vi "Main.vi"() -> ()   [LabVIEW 2026]
doc: "This template is for the Queued Message Handler design pattern.\n\nThe Event Handling Loop generates messages based on user interface actions.\n\nThe Message Handling Loop processes messages generated by the Event Handling Loop, or by other messages. The messages are string values, so new messages can be added easily to the Message Cases case structure in the Message Handling Loop. Each message cluster can also provide an optional value for Message Data, which is a variant that can be converted to whatever message-specific data is required."
uses:
  controls/UI Data.ctl
  controls/State_Enum.ctl
  support/Message Queue/Enqueue Message (Single).vi
  <vilib>/Utility/error.llb/Error Cluster From Error Code.vi
  <vilib>/ErrorRing/Error Ring.xnode
  support/Message Queue/Message Queue.lvlib
  support/User Event - Stop/User Event - Stop.lvlib
panel:
  in  "Mode":bool
  out "Panel":cluster{"On LED":bool, "Buzzer":bool}
  in  "Door Sensor":bool
  out "Recipes":string[][](array[string])
  in  "Key Pad":T1
  out "Display":string="00:00"
  in  "Exit":bool
  # "Manual"
  # "Recipe"
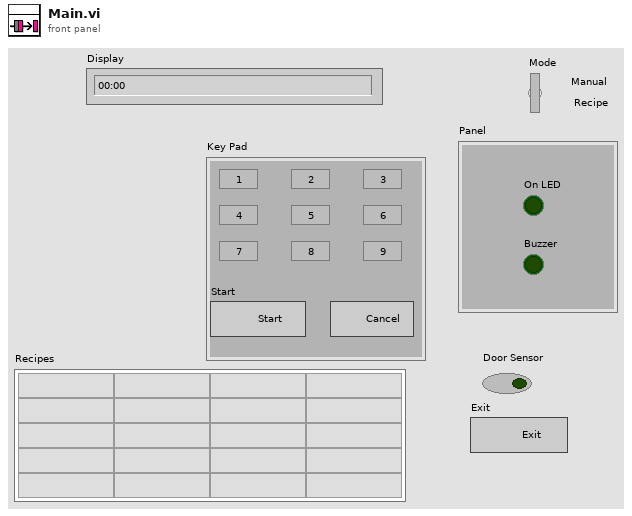
[diagram p1: front panel]
types:
  T1 = cluster{"1":bool, "2":bool, "3":bool, "4":bool, "5":bool, "6":bool, "7":bool, "8":bool, "9":bool, "Start":bool, "Cancel":bool}
  T2 = typedef "UI Data.ctl" = cluster{"Mode":bool, "Display":string, "Target Time ":dbl, "Data Display Ref":refnum<vi>, "Exit Button Ref":refnum<vi>, "Recipe":i32, "Step":i32, "Door Sensor":bool}
  T3 = typedef "Message Queue.lvlib/All Message Queues.ctl" = cluster{"UI":refnum<queue>}
  T4 = typedef "State_Enum.ctl" = enum16{"Complete", "Run", "Idle"}
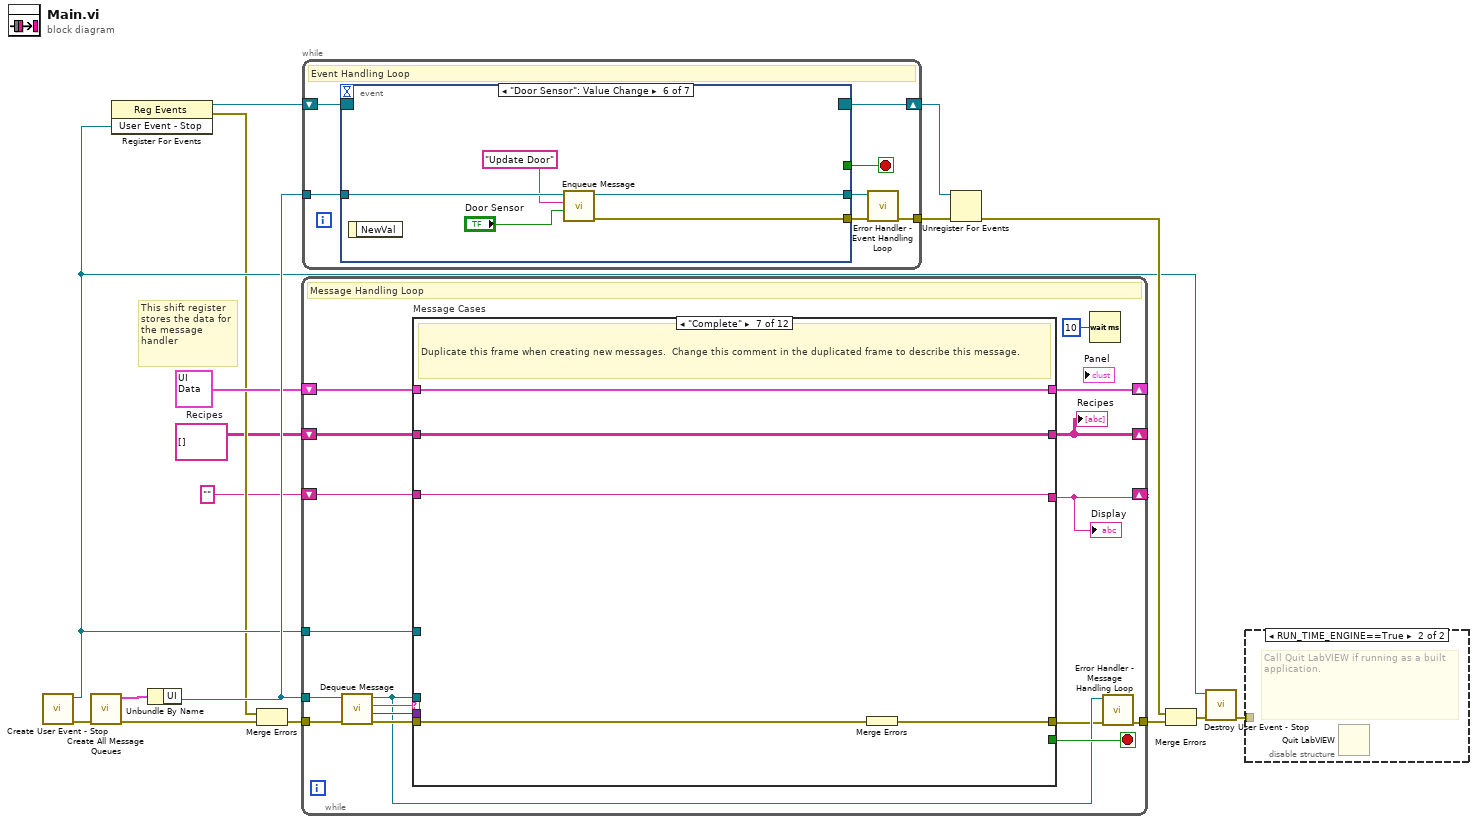
[diagram p0: block diagram]
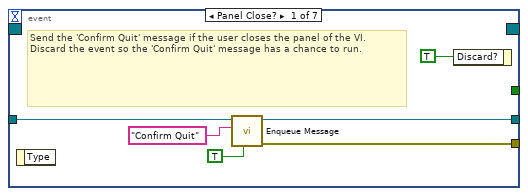
[diagram p3: hidden frame]
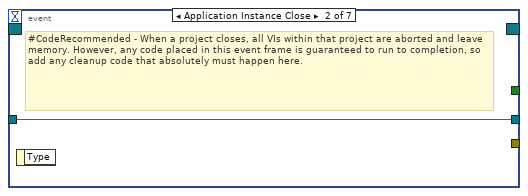
[diagram p4: hidden frame]
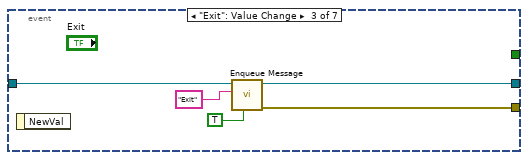
[diagram p5: hidden frame]
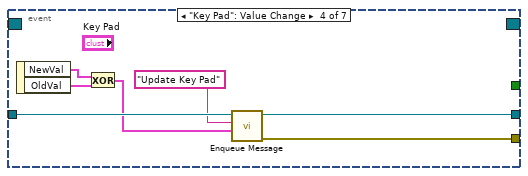
[diagram p6: hidden frame]
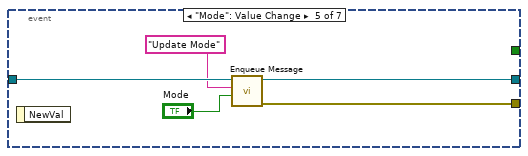
[diagram p7: hidden frame]
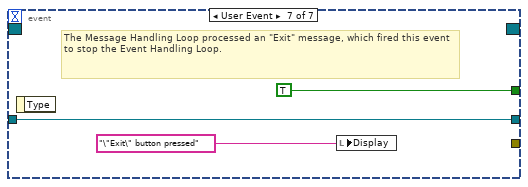
[diagram p8: hidden frame]
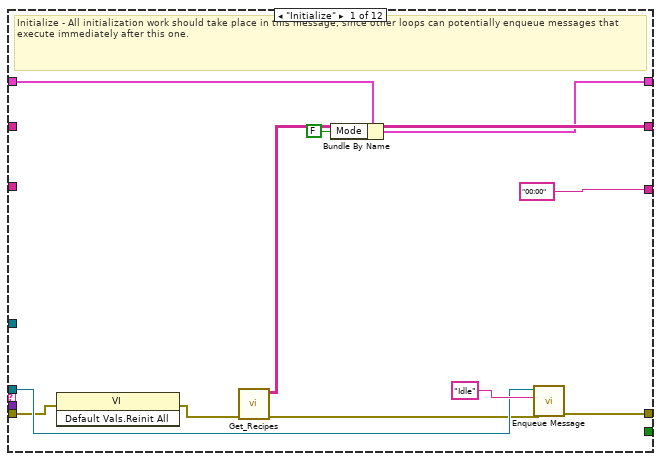
[diagram p9: hidden frame]
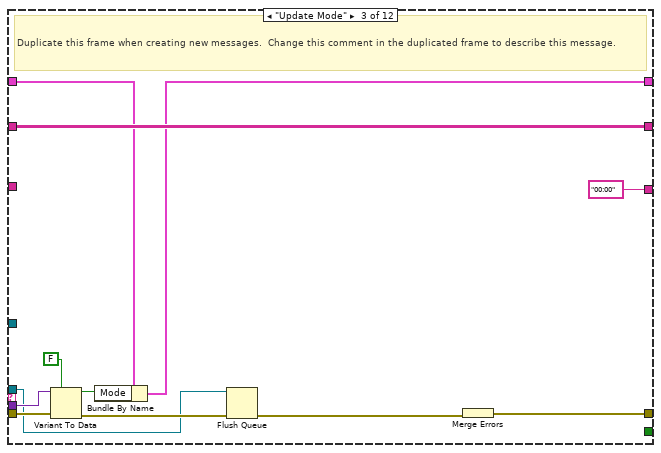
[diagram p11: hidden frame]
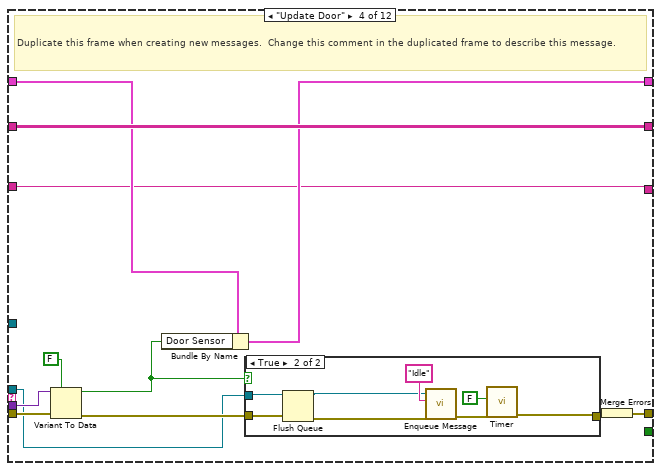
[diagram p12: hidden frame]
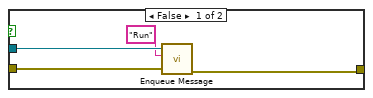
[diagram p13: hidden frame]
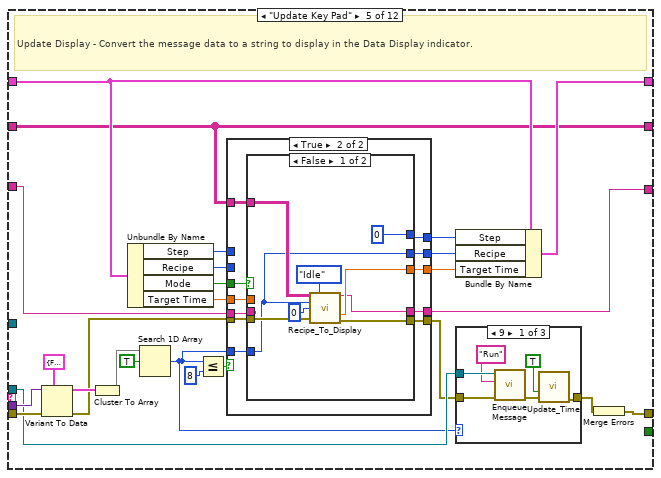
[diagram p14: hidden frame]
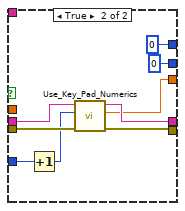
[diagram p16: hidden frame]
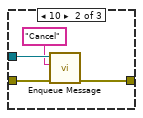
[diagram p17: hidden frame]
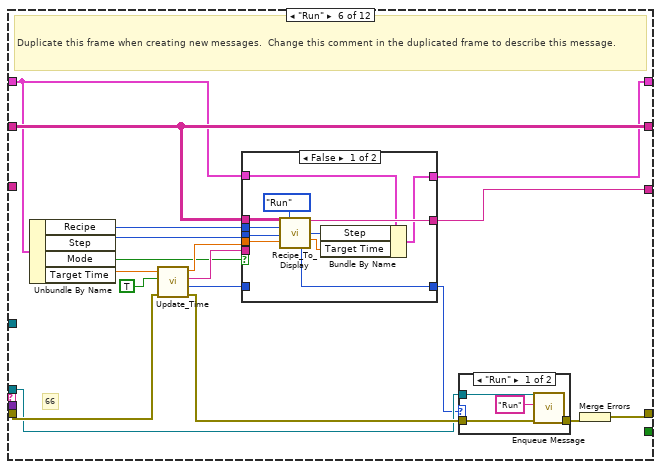
[diagram p19: hidden frame]
diagram:
  w2 = string[][] []  # Recipes
  # "This shift register stores the data for the message handler"
  n1 = call "Create User Event - Stop.vi"() -> ("error out"=w13:errorcluster, "User Event - Stop"=w5:refnum<user-event>)  [unwired: 10 in]
  n2 = call "Create All Message Queues.vi"("error in (no error)"=w13) -> ("error out"=w17:errorcluster, "Message Queues out"=w16:T3)  [unwired: 9 in]
  n3 = register-events(w5) -> (reference out=w6:refnum<event-registration>, error out=w3:errorcluster)  [unwired: 2 in]
  n4 = Unbundle By Name(w16) -> ("UI"=w14:refnum<queue>)
  n5 = Merge Errors(w3, w17) -> (w4:errorcluster)
  n6 = while {
    tunnel: w14 -> [w26]
    shift-right: [w33] -> _
    shift-left: T2 {"Mode"=FALSE, "Display"="", "Target Time "=0.0, "Data Display Ref"=refnum, "Exit Button Ref"=refnum, "Recipe"=0, "Step"=0, "Door Sensor"=FALSE} ("Data Cluster") -> [w34]
    tunnel: w5 -> [w31]
    tunnel: w4 -> [w30]
    tunnel: [w24] -> w15
    shift-right: [w22] -> _
    shift-left: w2 -> [w21]
    shift-right: [w19] -> _
    shift-left: "" ("String out") -> [w20]
    stop <- w32 stop-if-true
    # "Message Handling Loop"
    n7 = call "Dequeue Message.vi"("error in (no error)"=w30, "Message Queue"=w26) -> ("error out"=w29:errorcluster, "Message Data"=w27:variant, "Message"=w28:string, "dup Message Queue"=w25:refnum<queue>)  [unwired: 6 in]
    n8 = case "Message Cases" shown="\"Complete\"" w28 {
      selector: w28 -> [_ _ _ _ _ _ _ _ _ _ _ w240]
      tunnel: w25 -> [w43 _ w50 w63 w96 w169 _ _ w215 _ w237 _]
      tunnel: w29 -> [w41 w49 w59 w71 w110 w173 w201 w210 w219 w224 w230 _]
      tunnel: [w45 w49 w61 w73 w111 w174 w199 w204 w217 w222 w233 w241] -> w23
      tunnel: w34 -> [w37 w48 w57 w69 w101 w158 w200 w209 w218 w223 w236 w242]
      tunnel: [w36 w48 w55 w68 w102 w159 w200 w209 w218 w223 w236 w242] -> w33
      tunnel: [_ _ _ _ _ _ _ _ _ _ TRUE _] -> w32
      tunnel: w27 -> [_ _ w54 w67 w109 _ _ w208 _ _ w227 _]
      tunnel: w31 -> [_ _ _ _ _ _ _ _ _ _ w232 _]
      tunnel: [w39 w47 w60 w72 w93 w168 w198 w203 w212 w221 w226 w239] -> w22
      tunnel: w21 -> [_ w47 w60 w72 w93 w168 w198 w203 w212 w221 w226 w239]
      tunnel: ["00:00" ("Initial Message") w46 "00:00" ("String out") w66 w94 w157 w197 w202 w211 w220 w225 w238] -> w19
      tunnel: w20 -> [_ w46 _ w66 w103 _ w197 w202 w211 w220 w225 w238]
      frame "Initialize" {
        # "Initialize - All initialization work should take place in this message, since other loops can potentially enqueue messages that execute immediately after this one."
        n9 = invoke class="VI" method="Default Vals.Reinit All"(error in=w41) -> (error out=w42:errorcluster)  [unwired: 2 in, 2 out]
        n10 = call "Get_Recipes.vi"("error in (no error)"=w42) -> ("error out"=w40:errorcluster, "Recipes"=w39:string[][])  [unwired: 9 in]
        n11 = Bundle By Name(cluster=w37, "Mode"=FALSE) -> (w36:T2)
        n12 = call-poly "Enqueue Message.vi"("error in (no error)"=w40, "Message"="Idle", "Message Queue"=w43) -> ("error out"=w45:errorcluster)  [unwired: 7 in, 1 out]
      }
      frame "Idle" {
      }
      frame "Update Mode" {
        # "Duplicate this frame when creating new messages.  Change this comment in the duplicated frame to describe this message."
        n13 = Variant To Data(error in=w59, type=FALSE, Variant=w54) -> (data=w56:bool, error out=w52:errorcluster)
        n14 = Bundle By Name(cluster=w57, "Mode"=w56) -> (w55:T2)
        n15 = Flush Queue(queue=w50, error in (no error)=w52) -> (error out=w51:errorcluster)  [unwired: 2 out]
        n16 = Merge Errors(w51) -> (w61:errorcluster)
      }
      frame "Update Door" {
        # "Duplicate this frame when creating new messages.  Change this comment in the duplicated frame to describe this message."
        n17 = Variant To Data(error in=w71, type=FALSE, Variant=w67) -> (data=w62:bool, error out=w64:errorcluster)
        n18 = Bundle By Name(cluster=w69, "Door Sensor"=w62) -> (w68:T2)
        n19 = case shown="True" w62 {
          tunnel: [w76 w79] -> w65
          tunnel: w64 -> [w77 w84]
          tunnel: w63 -> [w75 w82]
          frame False {
            n20 = call-poly "Enqueue Message.vi"("error in (no error)"=w77, "Message"="Run", "Message Queue"=w75) -> ("error out"=w76:errorcluster)  [unwired: 7 in, 1 out]
          }
          frame True {
            n21 = Flush Queue(queue=w82, error in (no error)=w84) -> (queue out=w81:refnum<queue>, error out=w83:errorcluster)  [unwired: 1 out]
            n22 = call-poly "Enqueue Message.vi"("error in (no error)"=w83, "Message"="Idle", "Message Queue"=w81) -> ("error out"=w80:errorcluster)  [unwired: 7 in, 1 out]
            n23 = call "Timer.vi"("error in (no error)"=w80, "Advance?"=FALSE) -> ("error out"=w79:errorcluster)  [unwired: 6 in, 3 out]
          }
        }
        n24 = Merge Errors(w65) -> (w73:errorcluster)
      }
      frame "Update Key Pad" {
        # "Update Display - Convert the message data to a string to display in the Data Display indicator."
        n25 = Variant To Data(error in=w110, type=T1 {"1"=FALSE, "2"=FALSE, "3"=FALSE, "4"=FALSE, "5"=FALSE, "6"=FALSE, "7"=FALSE, "8"=FALSE, "9"=FALSE, "Start"=FALSE, "Cancel"=FALSE} ("x .xor. y?"), Variant=w109) -> (data=w107:T1, error out=w104:errorcluster)
        n26 = Cluster To Array(cluster=w107) -> (array=w106:bool[])
        n27 = Unbundle By Name(w101) -> ("Step"=w87:i32, "Recipe"=w86:i32, "Mode"=w100:bool, "Target Time"=w91:dbl)
        n28 = Search 1D Array(1D array=w106, element=TRUE) -> (index of element=w88:i32)  [unwired: 1 in]
        n29 = Less Or Equal?(x=w88, y=8) -> (x <= y?=w89:bool)
        n30 = case shown="True" w89 {
          tunnel: w104 -> [w116 w127]
          tunnel: w103 -> [w115 w126]
          tunnel: w100 -> [_ w125]
          tunnel: [w112 w124] -> w99
          tunnel: [w113 w123] -> w98
          tunnel: [w116 w122] -> w95
          tunnel: [w115 w121] -> w94
          tunnel: w93 -> [_ w120]
          tunnel: [w114 w119] -> w92
          tunnel: w91 -> [w114 w118]
          tunnel: w88 -> [_ w117]
          tunnel: w87 -> [w113 _]
          tunnel: w86 -> [w112 _]
          frame False {
          }
          frame True {
            n31 = case shown="False" w125 {
              tunnel: w127 -> [w135 w140]
              tunnel: w126 -> [_ w139]
              tunnel: [w128 0 ("upper limit")] -> w124
              tunnel: [0 0] -> w123
              tunnel: [w134 w143] -> w122
              tunnel: [w129 w142] -> w121
              tunnel: w120 -> [w133 _]
              tunnel: [w131 w141] -> w119
              tunnel: w118 -> [_ _]
              tunnel: w117 -> [w128 w137]
              frame False {
                n32 = call "Recipe_To_Display.vi"("Recipes"=w133, "State In"=State_Enum."Idle" ("Enum"), "Recipe"=w128, "Step In"=0 ("Step"), "error in (no error)"=w135) -> ("Display Out"=w129:string, "Target Time"=w131:dbl, "error out"=w134:errorcluster)  [unwired: 6 in, 2 out]
              }
              frame True {
                n33 = Increment(x=w137) -> (x+1=w138:i32)
                n34 = call "Use_Key_Pad_Numerics.vi"("error in (no error)"=w140, "Key Pad"=w138, "Display in"=w139) -> ("error out"=w143:errorcluster, "Elaspsed Time"=w141:dbl, "Display out"=w142:string)  [unwired: 6 in]
              }
            }
          }
        }
        n35 = Bundle By Name(cluster=w101, "Step"=w98, "Recipe"=w99, "Target Time"=w92) -> (w102:T2)
        n36 = case shown="9" w88 {
          tunnel: w96 -> [w151 w155 _]
          tunnel: [w148 w153 w156] -> w97
          tunnel: w95 -> [w146 w152 w156]
          frame 9 {
            n37 = call-poly "Enqueue Message.vi"("error in (no error)"=w146, "Message"="Run", "Message Queue"=w151) -> ("error out"=w149:errorcluster)  [unwired: 7 in, 1 out]
            n38 = call "Update_Time.vi"("error in (no error)"=w149, "Reset?"=TRUE) -> ("error out"=w148:errorcluster)  [unwired: 6 in, 3 out]
          }
          frame 10 {
            n39 = call-poly "Enqueue Message.vi"("error in (no error)"=w152, "Message"="Cancel", "Message Queue"=w155) -> ("error out"=w153:errorcluster)  [unwired: 7 in, 1 out]
          }
          frame 11, Default {
          }
        }
        n40 = Merge Errors(w97) -> (w111:errorcluster)
      }
      frame "Run" {
        # "66"
        # "Duplicate this frame when creating new messages.  Change this comment in the duplicated frame to describe this message."
        n41 = Unbundle By Name(w158) -> ("Recipe"=w167:i32, "Step"=w166:i32, "Mode"=w163:bool, "Target Time"=w172:dbl)
        n42 = call "Update_Time.vi"("error in (no error)"=w173, "Advance?"=TRUE, "Target Time"=w172) -> ("error out"=w171:errorcluster, "State"=w162:T4, "Display Out"=w164:string, "Time Remaining"=w165:dbl)  [unwired: 5 in]
        n43 = case shown="False" w163 {
          tunnel: w168 -> [w185 _]
          tunnel: w167 -> [w184 _]
          tunnel: w166 -> [w183 _]
          tunnel: w165 -> [w182 _]
          tunnel: [w180 w188] -> w157
          tunnel: w164 -> [_ w188]
          tunnel: w162 -> [_ w187]
          tunnel: [w179 w187] -> w161
          tunnel: [w175 w186] -> w159
          tunnel: w158 -> [w178 w186]
          frame False {
            n44 = call "Recipe_To_Display.vi"("Recipes"=w185, "State In"=State_Enum."Run" ("State"), "Recipe"=w184, "Step In"=w183, "Time Remaining"=w182) -> ("State Out"=w179:T4, "Display Out"=w180:string, "Step Out"=w177:i32, "Target Time"=w176:dbl)  [unwired: 6 in, 1 out]
            n45 = Bundle By Name(cluster=w178, "Step"=w177, "Target Time"=w176) -> (w175:T2)
          }
          frame True {
          }
        }
        n46 = case shown="\"Run\"" w161 {
          tunnel: w171 -> [w192 w196]
          tunnel: [w191 w195] -> w170
          tunnel: w169 -> [w189 w193]
          frame "Run" {
            n47 = call-poly "Enqueue Message.vi"("error in (no error)"=w192, "Message"="Run", "Message Queue"=w189) -> ("error out"=w191:errorcluster)  [unwired: 7 in, 1 out]
          }
          frame "Complete", Default {
            n48 = call-poly "Enqueue Message.vi"("error in (no error)"=w196, "Message"="Complete", "Message Queue"=w193) -> ("error out"=w195:errorcluster)  [unwired: 7 in, 1 out]
          }
        }
        n49 = Merge Errors(w170) -> (w174:errorcluster)
      }
      frame "Complete" {
        # "Duplicate this frame when creating new messages.  Change this comment in the duplicated frame to describe this message."
        n50 = Merge Errors(w201) -> (w199:errorcluster)
      }
      frame "Error" {
        # "Error - Display an error dialog. This message is sent by the \"Error Handler\" VIs at the end of other loops in this application."
        n51 = Variant To Data(error in=w210, type=errorcluster {"status"=FALSE, "code"=0, "source"=""} ("error constant"), Variant=w208) -> (data=w206:errorcluster, error out=w205:errorcluster)
        n52 = call <vilib>:"Simple Error Handler.vi"("error in (no error)"=w206) -> ()  [unwired: 4 in, 5 out]
        n53 = Merge Errors(w205) -> (w204:errorcluster)
      }
      frame "Confirm Quit" {
        # "#CodeNeeded - If you want to provide an \"Are you sure\" dialog (or some other notification) before the application exits, place that code here. This message is typically sent from a Panel Close? event."
        # "Confirm Quit - Message that can confirm whether or not the user wants to exit the application."
        n54 = call-poly "Enqueue Message.vi"("Priority Message? (F)"=TRUE, "error in (no error)"=w219, "Message"="Exit", "Message Queue"=w215) -> ("error out"=w216:errorcluster)  [unwired: 6 in, 1 out]
        n55 = Merge Errors(w216) -> (w217:errorcluster)
      }
      frame "---Copy This Frame---" {
        # "Duplicate this frame when creating new messages.  Change this comment in the duplicated frame to describe this message."
        n56 = Merge Errors(w224) -> (w222:errorcluster)
      }
      frame "Exit" {
        # "Stop the VI"
        # "Release the message queue reference"
        # "#CodeNeeded - Add any required cleanup code here. Note that if 'Exit' was called as a result of an error, an error dialog will be displayed. Add any custom error handling for an 'Exit' condition here as well."
        # "Exit - Exit the application."
        n57 = Variant To Data(type=errorcluster {"status"=FALSE, "code"=0, "source"=""} ("error constant"), Variant=w227) -> (data=w228:errorcluster)  [unwired: 1 in, 1 out]
        n58 = call <vilib>:"Simple Error Handler.vi"("error in (no error)"=w228) -> ()  [unwired: 4 in, 5 out]
        n59 = call "Fire User Event - Stop.vi"("User Event - Stop"=w232) -> ("error out"=w231:errorcluster)  [unwired: 10 in]
        n60 = Release Queue(queue=w237, error in (no error)=w230) -> (error out=w234:errorcluster)  [unwired: 1 in, 2 out]
        n61 = Merge Errors(w231, w234) -> (w233:errorcluster)
      }
      frame Default {
        # "'Default' case only runs if there is a message that isn't defined in any of the other cases.  Output a programming error."
        n62 = xnode "Error Ring"("parameter 0"=w240) -> ("error out"=w241:errorcluster)
      }
    }
    "Recipes" <- w22
    "Display" <- w19
    n63 = Wait (ms)(milliseconds to wait=u32 10) -> ()  [unwired: 1 out]
    n64 = call "Error Handler - Message Handling Loop.vi"("error in (no error)"=w23, "Message Queue"=w25) -> ("dup error in"=w24:errorcluster)  [unwired: 8 in, 1 out]
  }
  n65 = while {
    tunnel: w14 -> [w256]
    shift-right: [w254] -> w10
    shift-left: w6 -> [w255]
    tunnel: [w250] -> w7
    stop <- w252 stop-if-true
    # "Event Handling Loop"
    n66 = event shown="[5] \"Door Sensor\": Value Change" {
      selector: w255 -> [_ _ _ _ _ _ _]
      dyn-events: [_ _ _ _ _ _ _] -> w254
      timeout: _ -> [_ _ _ _ _ _ _]
      tunnel: [_ _ _ _ _ _ TRUE ("Discard?")] -> w252
      tunnel: w256 -> [w261 w263 w268 w273 w280 w285 w288]
      tunnel: [w260 _ w267 w271 w278 w283 _] -> w253
      tunnel: [w259 w263 w266 w272 w279 w284 w288] -> w251
      event Panel Close? {
        # "Send the 'Confirm Quit' message if the user closes the panel of the VI. Discard the event so the 'Confirm Quit' message has a chance to run."
        n67 = event-data() -> ()  [unwired: 1 in, 1 out]
        n68 = call-poly "Enqueue Message.vi"("Priority Message? (F)"=TRUE, "Message"="Confirm Quit", "Message Queue"=w261) -> ("error out"=w260:errorcluster, "dup Message Queue"=w259:refnum<queue>)  [unwired: 7 in]
        n69 = event-data("Discard?"=TRUE) -> ()  [unwired: 1 in, 1 out]
      }
      event Application Instance Close {
        # "#CodeRecommended - When a project closes, all VIs within that project are aborted and leave memory. However, any code placed in this event frame is guaranteed to run to completion, so add any cleanup code that absolutely must happen here."
        n70 = event-data() -> ()  [unwired: 1 in, 1 out]
      }
      event "Exit": Value Change {
        n71 = event-data() -> ()  [unwired: 1 in, 1 out]
        n72 = call-poly "Enqueue Message.vi"("Priority Message? (F)"=TRUE, "Message"="Exit", "Message Queue"=w268) -> ("error out"=w267:errorcluster, "dup Message Queue"=w266:refnum<queue>)  [unwired: 7 in]
      }
      event "Key Pad": Value Change {
        n73 = event-data() -> ("NewVal"=w275:T1, "OldVal"=w274:T1)  [unwired: 1 in]
        n74 = Exclusive Or(1:w274, 2:w275) -> (0:w269:T1)
        n75 = call-poly "Enqueue Message.vi"("Message Data"=w269, "Message"="Update Key Pad", "Message Queue"=w273) -> ("error out"=w271:errorcluster, "dup Message Queue"=w272:refnum<queue>)  [unwired: 7 in]
      }
      event "Mode": Value Change {
        n76 = event-data() -> ()  [unwired: 1 in, 1 out]
        n77 = call-poly "Enqueue Message.vi"("Message Data"="Mode", "Message"="Update Mode", "Message Queue"=w280) -> ("error out"=w278:errorcluster, "dup Message Queue"=w279:refnum<queue>)  [unwired: 7 in]
      }
      event "Door Sensor": Value Change {
        n78 = event-data() -> ()  [unwired: 1 in, 1 out]
        n79 = call-poly "Enqueue Message.vi"("Message Data"="Door Sensor", "Message"="Update Door", "Message Queue"=w285) -> ("error out"=w283:errorcluster, "dup Message Queue"=w284:refnum<queue>)  [unwired: 7 in]
      }
      event User Event {
        # "The Message Handling Loop processed an \"Exit\" message, which fired this event to stop the Event Handling Loop."
        n80 = event-data() -> ()  [unwired: 1 in, 1 out]
        n81 = local write "Display"("\"Exit\" button pressed" ("VI Stopped")) -> ()
      }
    }
    n82 = call "Error Handler - Event Handling Loop.vi"("error in (no error)"=w253, "Message Queue"=w251) -> ("dup error in"=w250:errorcluster)  [unwired: 8 in, 1 out]
  }
  n83 = Unregister For Events(event registration refnum=w10, error in=w7) -> (error out=w11:errorcluster)
  n84 = Merge Errors(w11, w15) -> (w12:errorcluster)
  n85 = call "Destroy User Event - Stop.vi"("error in (no error)"=w12, "User Event - Stop"=w5) -> ("error out"=w8:errorcluster)  [unwired: 9 in]
  n86 = disable-structure shown="RUN_TIME_ENGINE==True" {
    disable-tunnel: w8 -> [_ _]
    frame condition #0 (active) {
    }
    frame condition #1 {
      # "Call Quit LabVIEW if running as a built application."
      n87 = Quit LabVIEW() -> ()  [unwired: 1 in]
    }
  }
